vi "Panel.vi"(11 "InsertionPalettePanel in":refnum<class "InsertionPalettePanel.lvclass">) -> ()   [LabVIEW 2020, in "TSnax UI.lvlib" / "InsertionPalettePanel.lvclass"]
uses:
  InsertionPalettePanel.lvclass
  C:/Program Files (x86)/National Instruments/LabVIEW 2020/vi.lib/IlluminatedG/IG OOPanel/OOPanel/Panel/Panel.lvclass
  <vilib>/IlluminatedG/IG OOPanel/OOPanel/Panel/Basic UI State.ctl
  InsertionPalettePanel.lvclass/InsertionPalettePanel.ctl
  Drag Data Names.ctl
  <vilib>/IlluminatedG/IG OOPanel/OOPanel/Panel/Panel.lvclass
  <vilib>/IlluminatedG/IG OOPanel/OOPanel/OOPanel.lvlib
  TSnax UI.lvlib
panel:
  in  "InsertionList":string(tree)
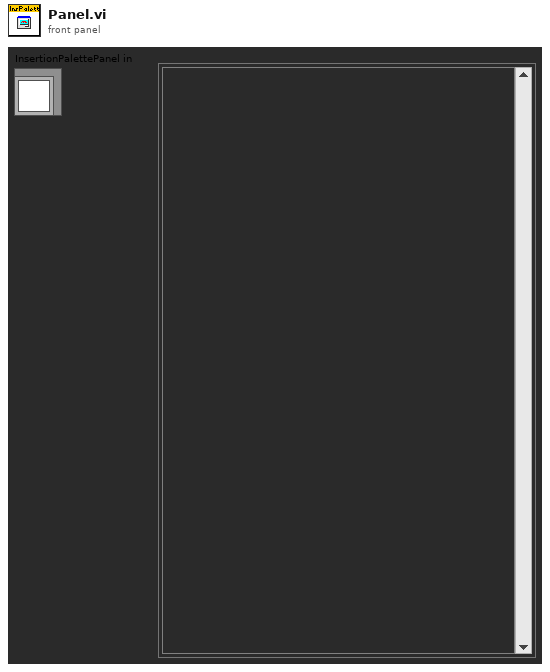
[diagram p1: front panel]
types:
  T1 = typedef "OOPanel.lvlib/Panel.lvclass/Basic UI State.ctl" = enum16{"Init", "Run", "Close"}
  T2 = typedef "TSnax UI.lvlib/Drag Data Names.ctl" = enum16{"TSnax_InsertStep"}
  T3 = typedef "OOPanel.lvlib/Panel.lvclass/Panel Events.ctl" = cluster{"Visbility":refnum<user-event>, "Close":refnum<user-event>}
  T4 = cluster{"Refresh Reg":refnum<event-registration>, "Event Registration Refnum":refnum<event-registration>}
  T5 = typedef "OOPanel.lvlib/Panel.lvclass/Visibility State.ctl" = enum16{"Idle", "Closed", "Hidden", "Visible", "Subpanel"}
  T6 = cluster{"data name":string, "drag data":variant}[]
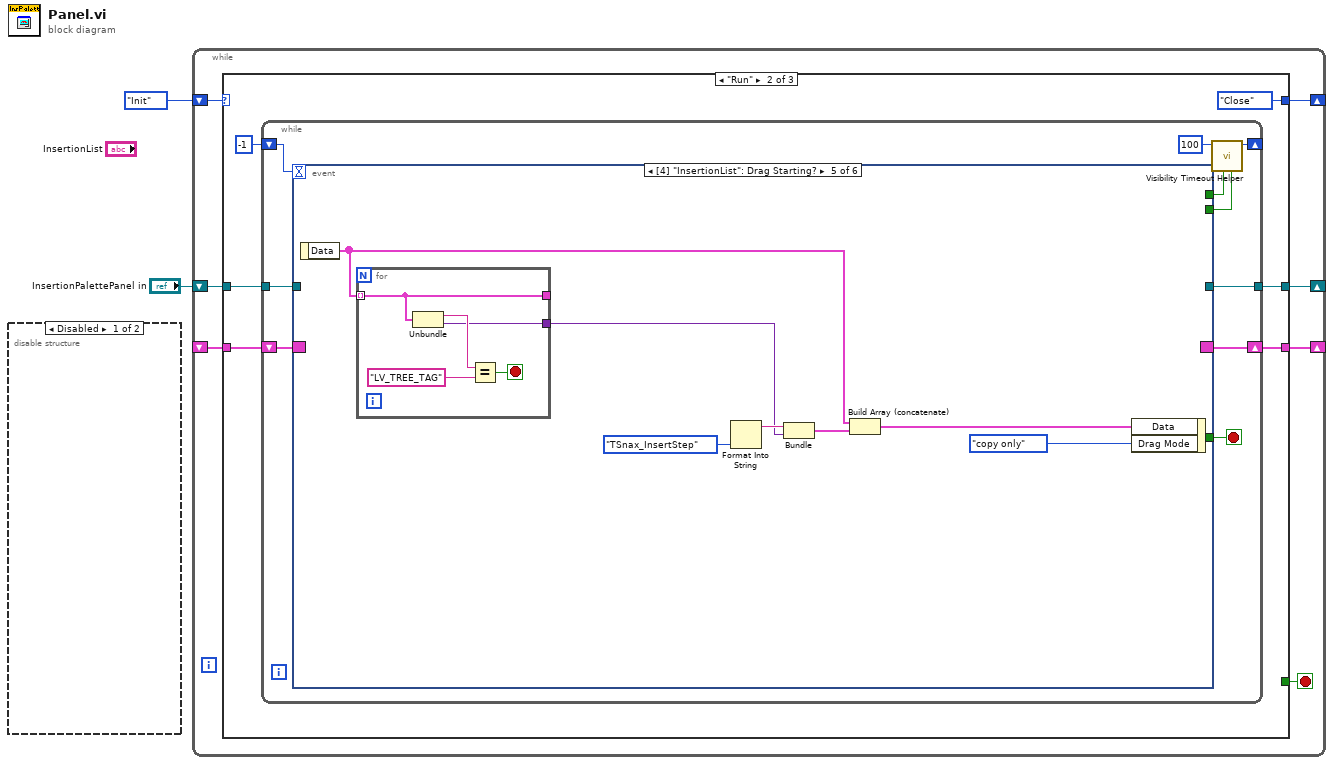
[diagram p0: block diagram]
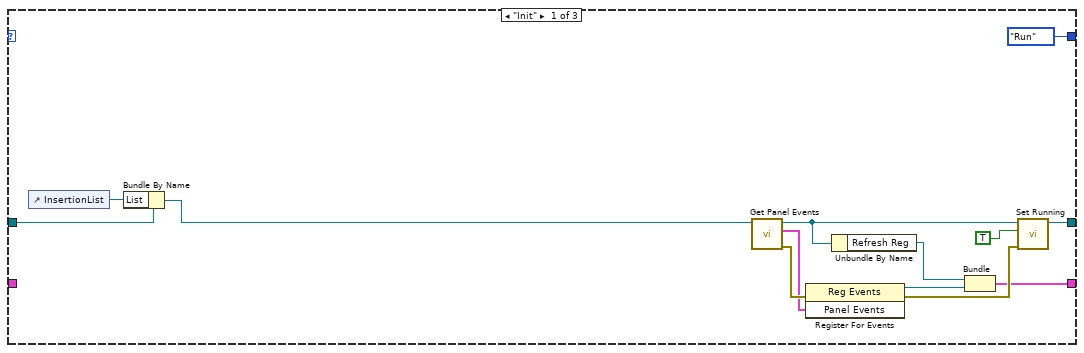
[diagram p3: hidden frame]
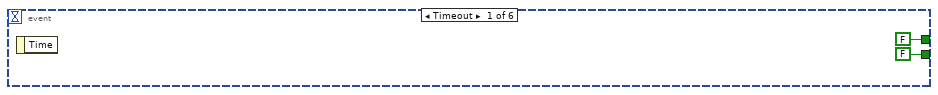
[diagram p4: hidden frame]
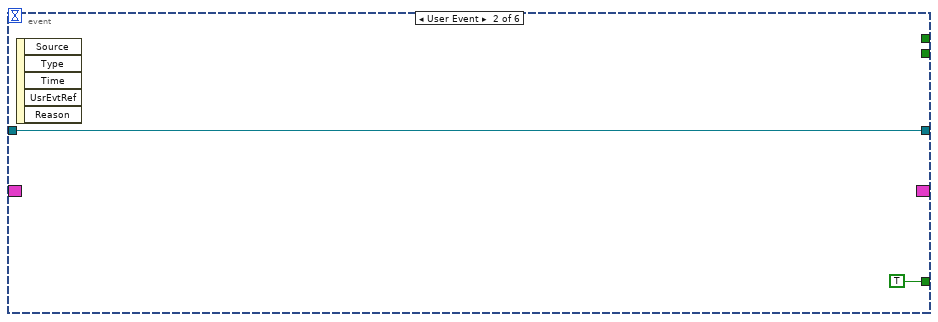
[diagram p5: hidden frame]
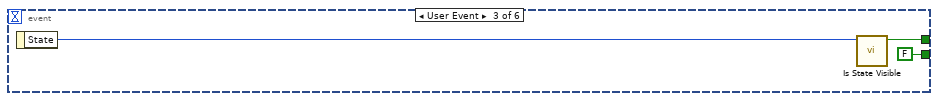
[diagram p6: hidden frame]
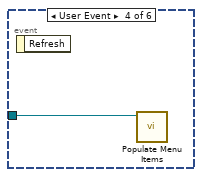
[diagram p7: hidden frame]
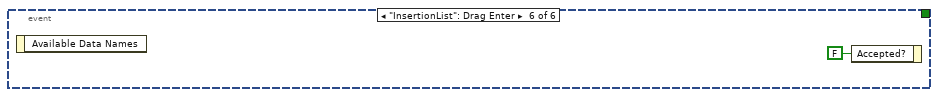
[diagram p8: hidden frame]
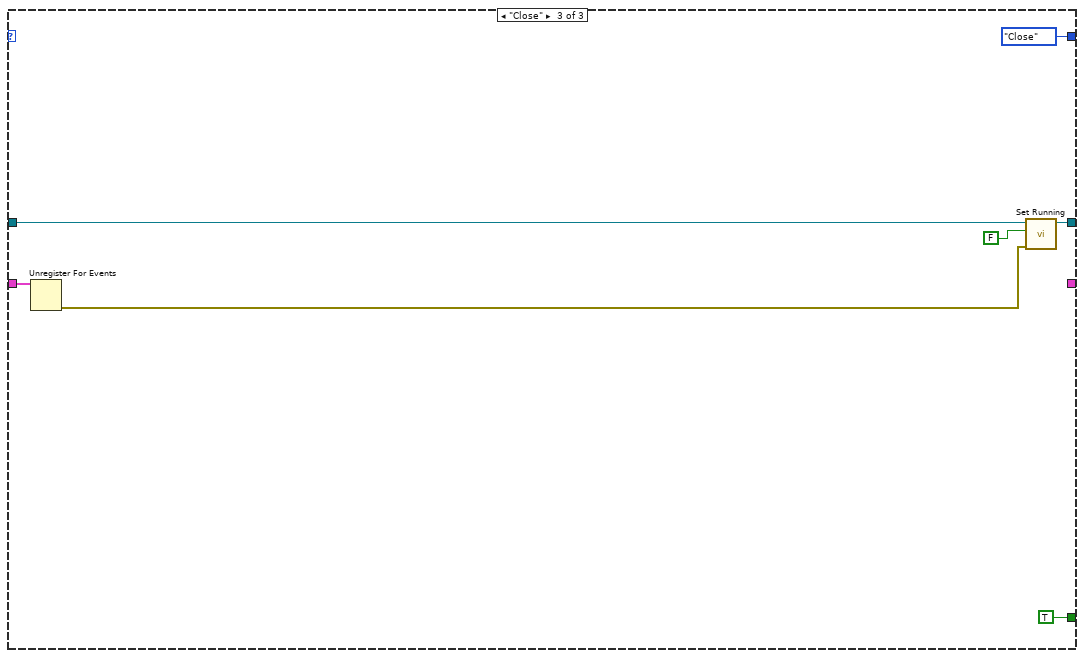
[diagram p9: hidden frame]
diagram:
  n1 = disable-structure shown="Disabled" {
    frame Disabled {
    }
    frame Enabled {
    }
  }
  n2 = while {
    shift-right: [w8] -> _
    shift-left: _ -> [w9]
    shift-right: [w6] -> _
    shift-left: Basic_UI_State."Init" ("Basic UI State") -> [w7]
    shift-right: [w4] -> _
    shift-left: "InsertionPalettePanel in" -> [w3]
    stop <- w5 stop-if-true
    n3 = case shown="\"Run\"" w7 {
      tunnel: w9 -> [_ w28 w62]
      tunnel: [w15 w26 _] -> w8
      tunnel: [Basic_UI_State."Run" ("Basic UI State") Basic_UI_State."Close" ("Basic UI State") Basic_UI_State."Close" ("Basic UI State")] -> w6
      tunnel: [_ _ TRUE] -> w5
      tunnel: [w17 w23 w60] -> w4
      tunnel: w3 -> [w10 w24 w61]
      frame "Init" {
        n4 = control-ref of="InsertionList"() -> (w12:refnum<vi>)
        n5 = Bundle By Name(cluster=w10, "List"=w12) -> (w11:refnum<class "InsertionPalettePanel.lvclass">)
        n6 = call <vilib>:"Get Panel Events.vi"("Panel in"=w11) -> ("error out"=w22:errorcluster, "Panel Events"=w19:T3, "Panel out"=w14:refnum<class "InsertionPalettePanel.lvclass">)  [unwired: 8 in]
        n7 = register-events(error in=w22, w19) -> (reference out=w16:refnum<event-registration>, error out=w20:errorcluster)  [unwired: 1 in]
        n8 = Unbundle By Name(w14) -> ("Refresh Reg"=w13:refnum<event-registration>)
        n9 = Bundle("Refresh Reg"=w13, "Event Registration Refnum"=w16) -> (w15:T4)  [unwired: 1 in]
        n10 = call <vilib>:"Set Running.vi"("error in (no error)"=w20, "Running"=TRUE, "Panel in"=w14) -> ("Panel out"=w17:refnum<class "InsertionPalettePanel.lvclass">)  [unwired: 7 in, 1 out]
      }
      frame "Run" {
        n11 = while {
          shift-right: [w34] -> w26
          shift-left: w28 -> [w35]
          shift-right: [w37] -> _
          shift-left: -1 ("Timeout") -> [w36]
          tunnel: w24 -> [w30]
          tunnel: [w29] -> w23
          stop <- w31 stop-if-true
          n12 = event shown="[4] \"InsertionList\": Drag Starting?" {
            selector: w35 -> [_ _ _ _ _ _]
            dyn-events: [_ _ _ _ _ _] -> w34
            timeout: w36 -> [_ _ _ _ _ _]
            tunnel: [FALSE _ w44 _ _ _] -> w33
            tunnel: [FALSE _ FALSE _ _ _] -> w32
            tunnel: [_ TRUE _ _ _ _] -> w31
            tunnel: w30 -> [_ w41 _ w46 _ _]
            tunnel: [_ w41 _ _ _ _] -> w29
            event Timeout {
              n13 = event-data() -> ()  [unwired: 1 in, 1 out]
            }
            event User Event {
              n14 = event-data() -> ()  [unwired: 1 in, 5 out]
            }
            event User Event {
              n15 = event-data() -> ("State"=w45:T5)  [unwired: 1 in]
              n16 = call <vilib>:"Is State Visible.vi"("Visibility"=w45) -> ("Visible"=w44:bool)  [unwired: 10 in]
            }
            event User Event {
              n17 = event-data() -> ()  [unwired: 1 in, 1 out]
              n18 = call "Populate Menu Items.vi"("InsertionPalettePanel in"=w46) -> ()  [unwired: 9 in, 2 out]
            }
            event "InsertionList": Drag Starting? {
              n19 = event-data() -> ("Data"=w48:T6)  [unwired: 1 in]
              n20 = for {
                tunnel: w48 -> [w57] mode=indexing
                tunnel: [w57] -> _
                tunnel: [w54] -> w47
                stop <- w56 stop-if-true
                n21 = Unbundle(w57) -> ("data name"=w55:string, "drag data"=w54:variant)
                n22 = Equal?(x=w55, y="LV_TREE_TAG") -> (x = y?=w56:bool)
              }
              n23 = Format Into String(Drag_Data_Names."TSnax_InsertStep" ("Drag Data Names")) -> (resulting string=w52:string)  [unwired: 3 in, 1 out]
              n24 = Bundle(w52, "drag data"=w47) -> (w51:cluster{string, "drag data":variant})  [unwired: 1 in]
              n25 = Build Array (concatenate)(w48, w51) -> (w50:T6)
              n26 = event-data("Data"=w50, "Drag Mode"=enum32{"copy or move", "copy only", "move only"}."copy only") -> ()  [unwired: 1 in, 1 out]
            }
            event "InsertionList": Drag Enter {
              n27 = event-data() -> ()  [unwired: 1 in, 1 out]
              n28 = event-data("Accepted?"=FALSE) -> ()  [unwired: 1 in, 1 out]
            }
          }
          n29 = call <vilib>:"Visibility Timeout Helper.vi"("Update?"=w32, "Use Timeout?"=w33, "Visible Timeout mS"=100) -> ("Timeout"=w37:i32)  [unwired: 8 in]
        }
      }
      frame "Close" {
        n30 = Unregister For Events(event registration refnum=w62) -> (error out=w64:errorcluster)  [unwired: 1 in]
        n31 = call <vilib>:"Set Running.vi"("error in (no error)"=w64, "Running"=FALSE, "Panel in"=w61) -> ("Panel out"=w60:refnum<class "InsertionPalettePanel.lvclass">)  [unwired: 7 in, 1 out]
      }
    }
  }
